vi "CSC_QuadPlanner.vi"(6 "F range":cluster{"Fmin":dbl, "Fmax":dbl}, 7 "TargetF(N)":dbl format="%#_13g", 8 "error in (no error)":errorcluster, 9 "LockedJoint(StartFrom0)":i32[](array[numeric]), 10 "DesireTorque(Nm)":dbl[](array[numeric]), 11 "C-Alex in":refnum<class "CableSerialChain.lvclass">) -> (0 "error out":errorcluster, 1 "Jacobian for Cables":T1, 2 "Planned Tension":dbl[](array[numeric]), 3 "C-Alex out":refnum<class "CableSerialChain.lvclass">, 4 "Solved":bool)   [LabVIEW 2015, in "CableSerialChain.lvclass"]
uses:
  CableSerialChain.lvclass
  <vilib>/Analysis/Matrix/Datatypes/RealMatrix.ctl
  <vilib>/gmath/NumericalOptimization/stopping criteria.ctl
  CableSerialChain.lvclass/CableSerialChain.ctl
  <vilib>/Analysis/7linalg.llb/Create Special Real Matrix.vi
  <vilib>/Analysis/Matrix/Numeric/Conversions/Matrix To Array - RM.vi
  <vilib>/gmath/NumericalOptimization/Quadratic Programming AS.vi
  <vilib>/gmath/NI_Gmath.lvlib
  <vilib>/Analysis/NI_AALPro.lvlib
  <vilib>/Analysis/Matrix/NI_Matrix.lvlib
panel:
  out "Torque":dbl[](array[numeric])
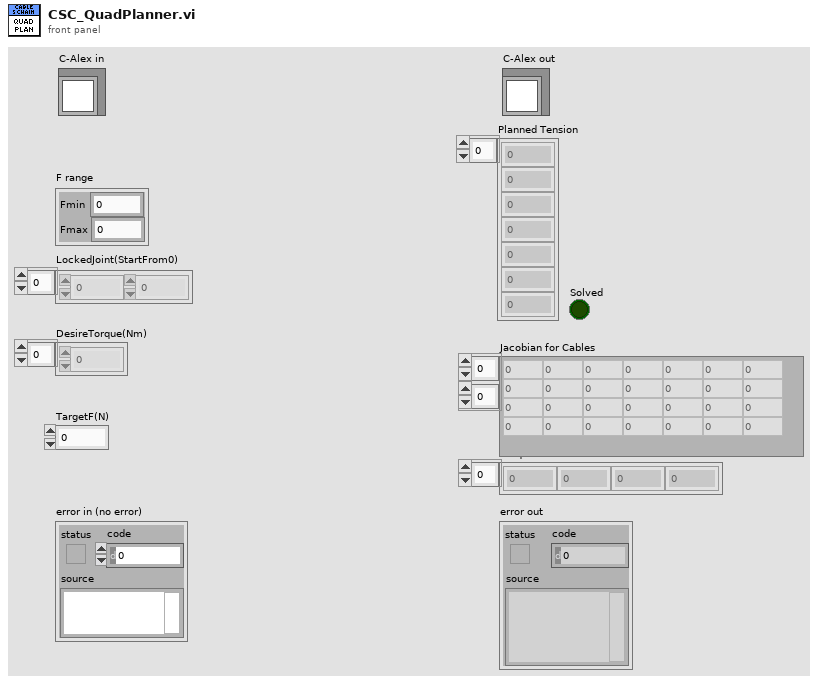
[diagram p1: front panel]
types:
  T1 = typedef "NI_Matrix.lvlib/RealMatrix.ctl" = dbl[][]
  T2 = typedef "NI_Gmath.lvlib/stopping criteria.ctl" = cluster{"function tolerance":dbl, "parameter tolerance":dbl, "max iterations":i32, "max function calls":i32, "gradient tolerance":dbl, "max time (sec)":dbl}
  T3 = typedef "CableSerialChain.lvclass/Cable.ctl" = cluster{"RoutingPtsInLCS":T4[], "Cable ID":i32, "ActiveSegments":i32[][]}
  T4 = typedef "Bodies.lvclass/PointOnBody.ctl" = cluster{"Coord4":dbl[], "ID":i32}
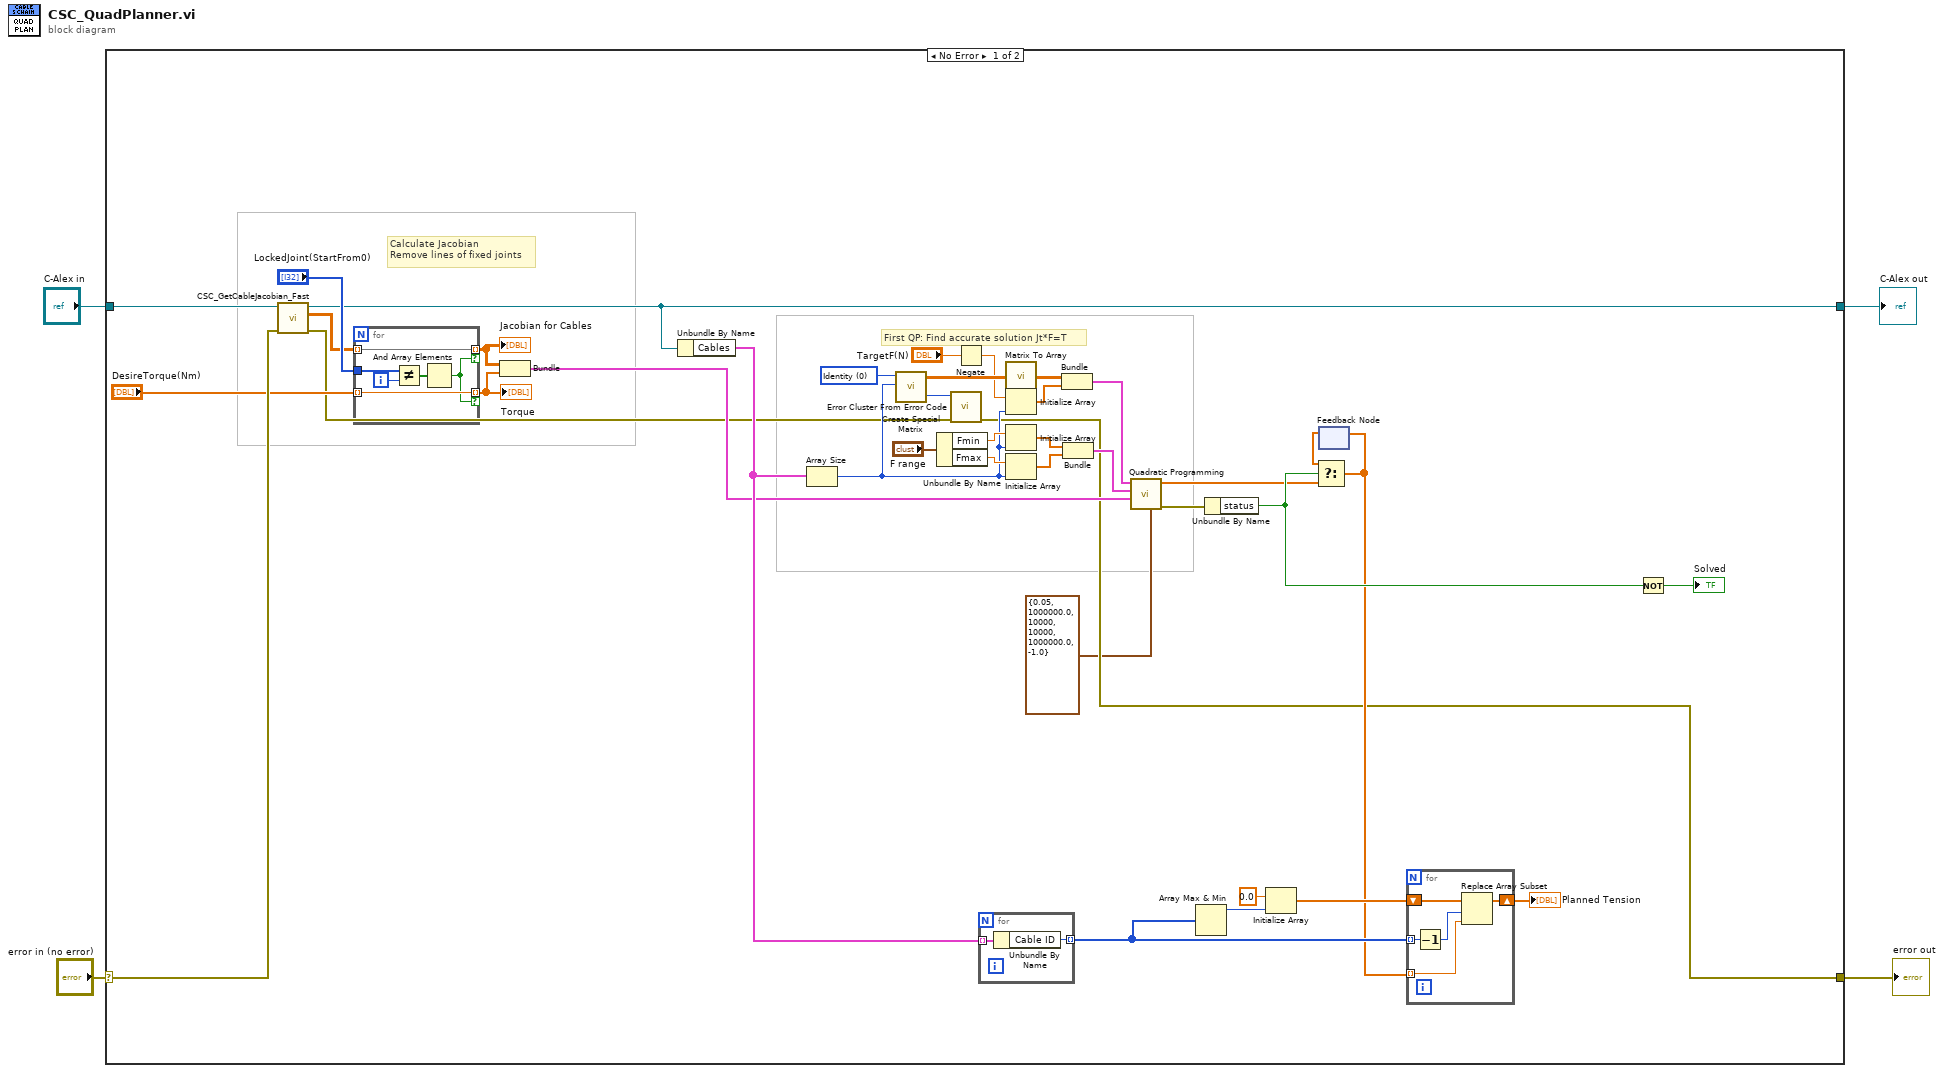
[diagram p0: block diagram]
diagram:
  n1 = case shown="No Error" "error in (no error)" {
    selector: "error in (no error)" -> [w17 w57]
    tunnel: [w9 w57] -> w3
    tunnel: [w14 w58] -> w1
    tunnel: "C-Alex in" -> [w19 w58]
    frame No Error {
      w38 = 0 items=["Identity", "Diagonal", "Toeplitz", "Vandermonde", "Companion", "Hankel", "Hadamard", "Wilkinson", "Hilbert", "Inverse Hilbert", "Rosser", "Pascal"] ("matrix type")
      # "First QP: Find accurate solution Jt*F=T"
      # "Calculate Jacobian\nRemove lines of fixed joints"
      n2 = call "CSC_GetCableJacobian_Fast.vi"("error in (no error)"=w17, "C-Alex in"=w19) -> ("error out"=w13:errorcluster, "Jacobian for Cables"=w28:T1, "C-Alex out"=w14:refnum<class "CableSerialChain.lvclass">)  [unwired: 7 in]
      n3 = for {
        tunnel: "LockedJoint(StartFrom0)" -> [w55]
        tunnel: w28 -> [w53] mode=indexing
        tunnel: "DesireTorque(Nm)" -> [w52] mode=indexing
        tunnel: [w53] -> w27 mode=indexing if=w51
        tunnel: [w52] -> w26 mode=indexing if=w51
        i -> [w56]
        n4 = Not Equal?(x=w55, y=w56) -> (x != y?=w54:bool[])
        n5 = And Array Elements(Boolean array=w54) -> (logical AND=w51:bool)
      }
      "Torque" <- w26
      "Jacobian for Cables" <- w27
      n6 = Bundle("Jacobian for Cables"=w27, w26) -> (w15:cluster{"Jacobian for Cables":dbl[][], dbl[]})  [unwired: 1 in]
      n7 = Unbundle By Name(w14) -> ("Cables"=w18:T3[])
      n8 = Array Size(array=w18) -> (size(s)=w31:i32)
      n9 = call-poly <vilib>:"Create Special Matrix.vi"("matrix type"=w38, "matrix size"=w31) -> ("Special Matrix"=w37:T1, "error"=w34:i32)  [unwired: 3 in]
      n10 = Unbundle By Name("F range") -> ("Fmin"=w42:dbl, "Fmax"=w41:dbl)
      n11 = call <vilib>:"Error Cluster From Error Code.vi"("error in (no error)"=w13, "error code (0)"=w34) -> ("error out"=w9:errorcluster)  [unwired: 7 in]
      n12 = Negate(x="TargetF(N)") -> (-x=w6:dbl)
      n13 = for {
        tunnel: w18 -> [w50] mode=indexing
        tunnel: [w49] -> w24 mode=indexing
        n14 = Unbundle By Name(w50) -> ("Cable ID"=w49:i32)
      }
      n15 = call-poly <vilib>:"Matrix To Array.vi"("Real Matrix"=w37) -> ("Real 2D Array"=w36:dbl[][])
      n16 = Initialize Array(w6, w31) -> (w29:dbl[])
      n17 = Initialize Array(w42, w31) -> (w33:dbl[])
      n18 = Initialize Array(w41, w31) -> (w40:dbl[])
      n19 = Bundle("Real 2D Array"=w36, w29) -> (w35:cluster{"Real 2D Array":dbl[][], dbl[]})  [unwired: 1 in]
      n20 = Bundle(w33, w40) -> (w39:cluster{dbl[], dbl[]})  [unwired: 1 in]
      n21 = call-poly <vilib>:"Quadratic Programming.vi"("stopping criteria"=T2 {"function tolerance"=0.05, "parameter tolerance"=1000000.0, "max iterations"=10000, "max function calls"=10000, "gradient tolerance"=1000000.0, "max time (sec)"=-1.0}, "equality constraints"=w15, "parameter bounds"=w39, "objective function"=w35) -> ("error out"=w8:errorcluster, "minimum"=w12:dbl[])  [unwired: 4 in, 2 out]
      n22 = Array Max & Min(array=w24) -> (max value=w23:i32)  [unwired: 3 out]
      n23 = Unbundle By Name(w8) -> ("status"=w22:bool)
      n24 = Initialize Array(0.0 ("element"), w23) -> (w21:dbl[])
      n25 = feedback #1() -> (w5:dbl[])  [unwired: 1 in]
      n26 = Select(t=w5, s=w22, f=w12) -> (s? t:f=w11:dbl[])
      n27 = feedback-in #1(w11) -> ()
      n28 = for {
        tunnel: w24 -> [w48] mode=indexing
        shift-right: [w46] -> w10
        shift-left: w21 -> [w45]
        tunnel: w11 -> [w44] mode=indexing
        n29 = Decrement(x=w48) -> (x-1=w47:i32)
        n30 = Replace Array Subset(array=w45, new element=w44, index=w47) -> (w46:dbl[])
      }
      "Planned Tension" <- w10
      n31 = Not(x=w22) -> (.not. x?=→"Solved":bool)
    }
    frame Error {
    }
  }
  "error out" <- w3
  "C-Alex out" <- w1
